vi "DestroyBroadcastEvents.vi"(8 "error in (no error)":errorcluster) -> (0 "error out":errorcluster)   [LabVIEW 2018, in "AcPwrPlugins.lvlib"]
doc: "This VI destroys all the events that are used to broadcast messages from the Main.vi."
uses:
  AcPwrPlugins.lvlib
  AcPwrShared/AcPwrBroadcastEvents.ctl
  AcPwrShared/clEventType.ctl
  AcPwrShared/AcPwrShared.lvlib
panel:
  out "clAcPwrEvents":T1
  # "If you want to add another Broadcast Events, open this typedef, copy an existing event and rename it to your event name.\n\nNext create an \"arg\" typedef for the  data and put it into PublicAPI/Arguments/Broadcasts\n\nAfter that, you will need to create a new roadcast vi in Protected/Broadcast.  Look at DidInit.vi or the reportError.vi as examples."
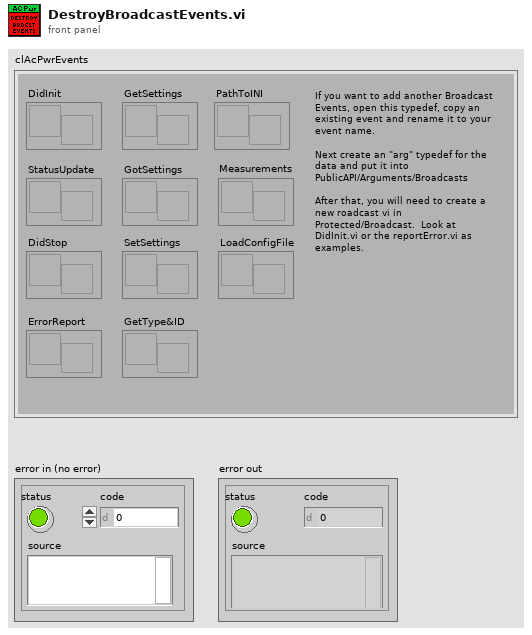
[diagram p1: front panel]
types:
  T1 = typedef "AcPwrShared.lvlib/AcPwrBroadcastEvents.ctl" = cluster{"DidInit":refnum<user-event>, "StatusUpdate":refnum<user-event>, "ErrorReport":refnum<user-event>, "DidStop":refnum<user-event>, "PathToINI":refnum<user-event>, "Measurements":refnum<user-event>, "LoadConfigFile":refnum<user-event>, "GetSettings":refnum<user-event>, "SetSettings":refnum<user-event>, "GetType&ID":refnum<user-event>, "GotSettings":refnum<user-event>}
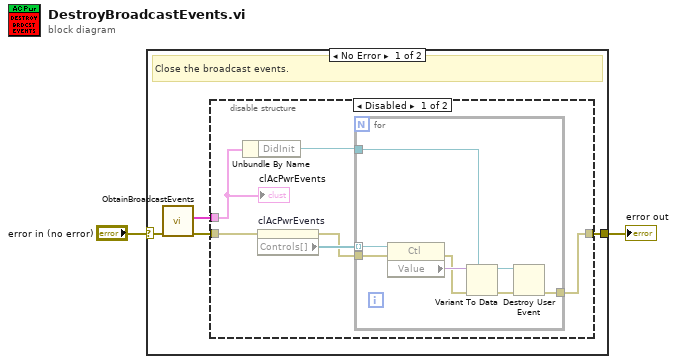
[diagram p0: block diagram]
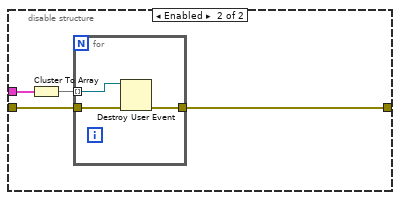
[diagram p2: hidden frame]
diagram:
  n1 = case shown="No Error" "error in (no error)" {
    selector: "error in (no error)" -> [w5 w28]
    tunnel: [w6 w28] -> w2
    frame No Error {
      # "Close the broadcast events."
      n2 = call "ObtainBroadcastEvents.vi"("error in (no error)"=w5) -> ("error out"=w4:errorcluster, "clAcPwrEvents"=w3:T1)  [unwired: 9 in]
      n3 = disable-structure shown="Disabled" {
        disable-tunnel: [w12 w21] -> w6
        disable-tunnel: w4 -> [w10 w23]
        disable-tunnel: w3 -> [w8 w24]
        frame Disabled {
          n4 = Unbundle By Name(w8) -> ("DidInit"=w7:refnum<user-event>)
          n5 = property on="clAcPwrEvents" class="Clust (strict)"(error in=w10) -> (error out=w9:errorcluster, "Controls[]"=w11:refnum<vi>[])  [unwired: 1 in, 1 out]
          n6 = for {
            tunnel: w11 -> [w20] mode=indexing
            tunnel: w9 -> [w15]
            tunnel: [w17] -> w12
            tunnel: w7 -> [w13]
            n7 = property class="Ctl"(reference=w20, error in=w15) -> (error out=w14:errorcluster, "Value"=w19:variant)  [unwired: 1 out]
            n8 = Variant To Data(error in=w14, type=w13, Variant=w19) -> (data=w16:refnum<user-event>, error out=w18:errorcluster)
            n9 = Destroy User Event(user event=w16, error in=w18) -> (error out=w17:errorcluster)
          }
          "clAcPwrEvents" <- w8
        }
        frame Enabled {
          n10 = Cluster To Array(cluster=w24) -> (array=w22:refnum<user-event>[])
          n11 = for {
            tunnel: [w27] -> w21
            tunnel: w23 -> [w26]
            tunnel: w22 -> [w25] mode=indexing
            n12 = Destroy User Event(user event=w25, error in=w26) -> (error out=w27:errorcluster)
          }
        }
      }
    }
    frame Error {
    }
  }
  "error out" <- w2
